vi "P-733 Control.vi"(0 "P-733 Notifier":refnum<notifier>, 5 "Stage Actions":T1={"Action"=enum."Get Position", "Axis"=[], "Setpoint"=[], "Velocity"=0.5, "Cmd Recvd?"=FALSE, "Position"=[], "Status"=enum."Error", "Misc"=variant} {"Velocity" min=0.0 max=1.0 step=0.01}, 11 "VISA In":refnum<visa-resource-name>, 13 "Axis Names":string[](array[string])) -> (4 "P-612 Notifier (Dup)":refnum<notifier>)   [LabVIEW 2016]
uses:
  Stages Controls/Stage Notifier Element.ctl
  Stages Controls/Stage Actions.ctl
  Stages Controls/Stage Status.ctl
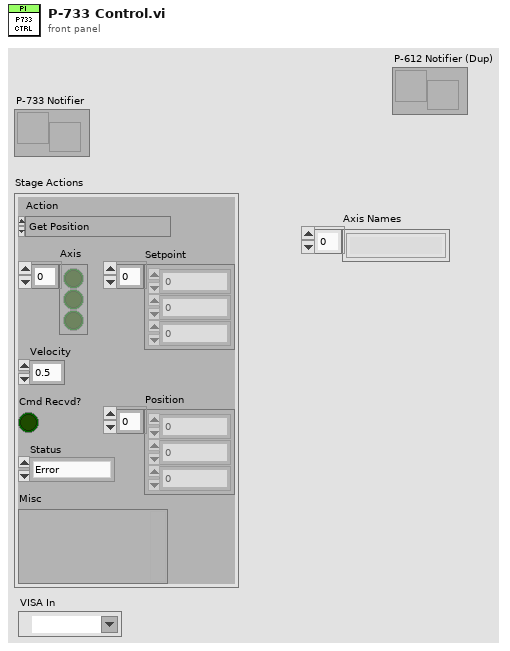
[diagram p1: front panel]
types:
  T1 = typedef "Stage Notifier Element.ctl" = cluster{"Action":T2, "Axis":bool[], "Setpoint":dbl[], "Velocity":dbl, "Cmd Recvd?":bool, "Position":dbl[], "Status":T3, "Misc":variant}
  T2 = typedef "Stage Actions.ctl" = enum16{"Get Position", "MVR", "MOVE", "HALT", "ONTARGET", "ERROR", "REFERENCE", "INIT", "VELOCITY", "STATUS", "EXIT", "HOME", "ZEROPOS", "NANOPOS", "ANALOG", "QUIT"}
  T3 = typedef "Stage Status.ctl" = enum16{"Error", "Abort", "Busy", "On Target"}
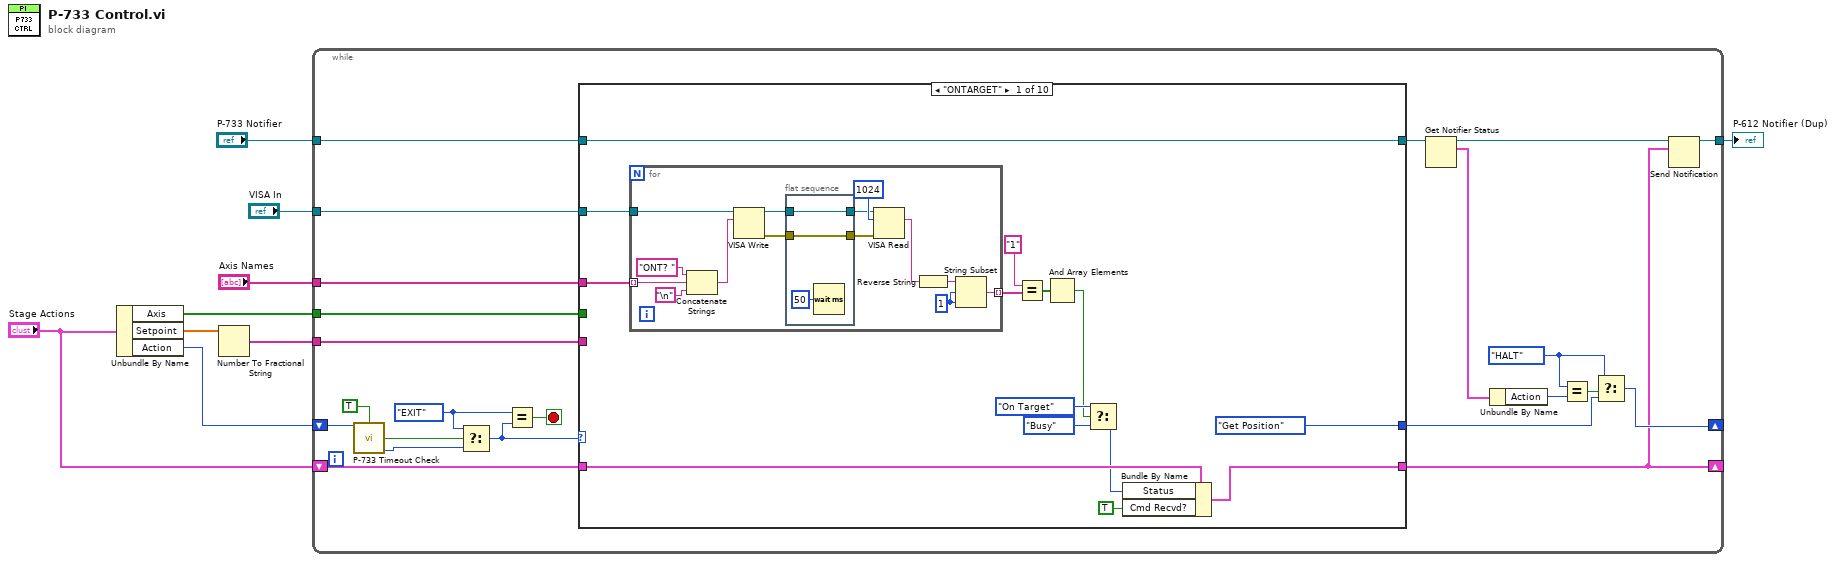
[diagram p0: block diagram]
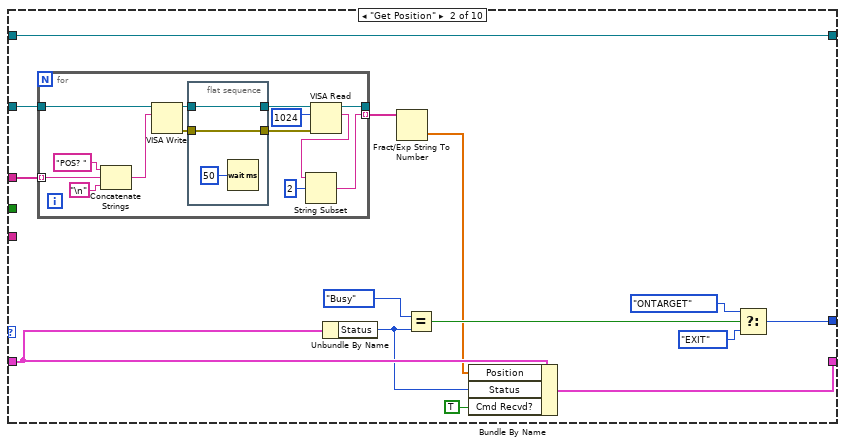
[diagram p2: hidden frame]
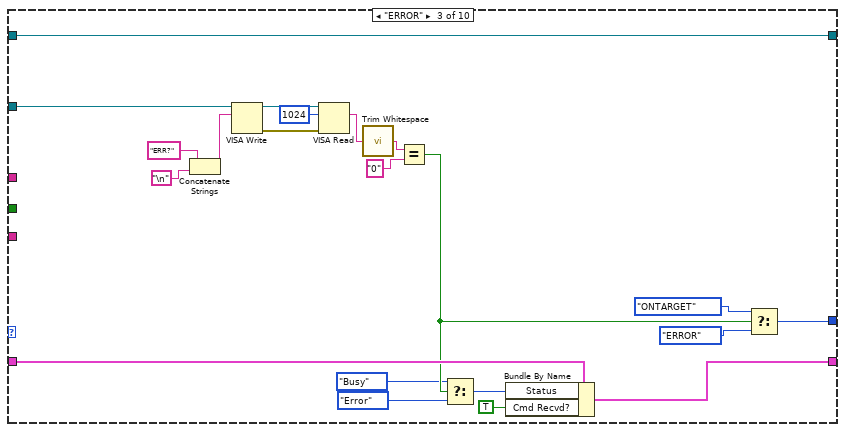
[diagram p3: hidden frame]
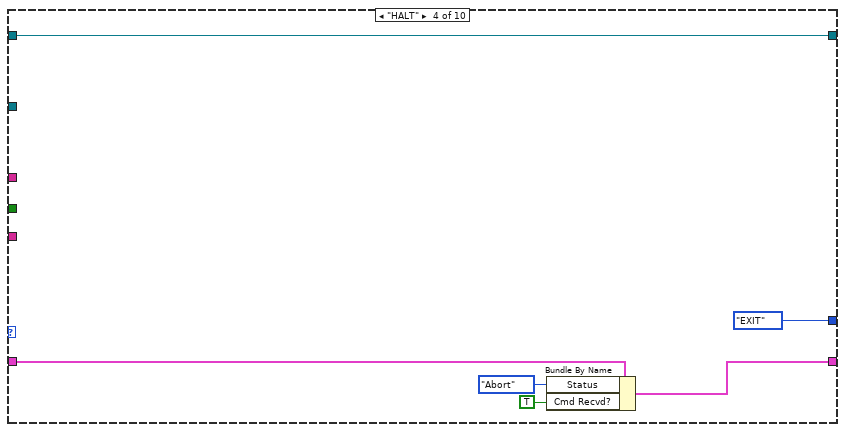
[diagram p4: hidden frame]
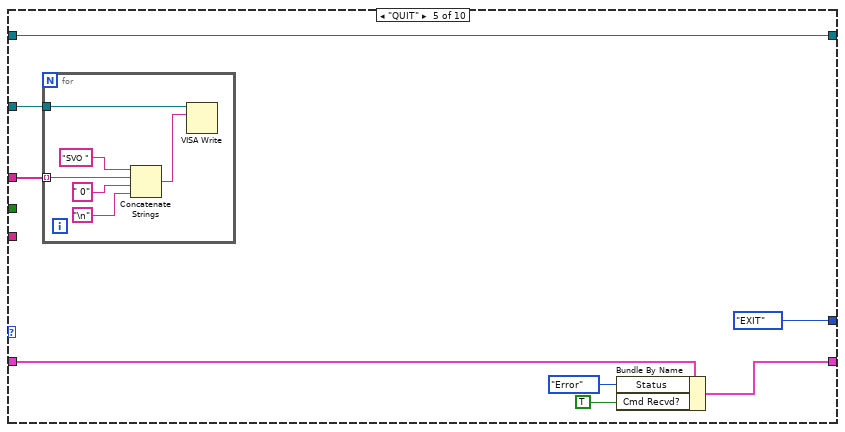
[diagram p5: hidden frame]
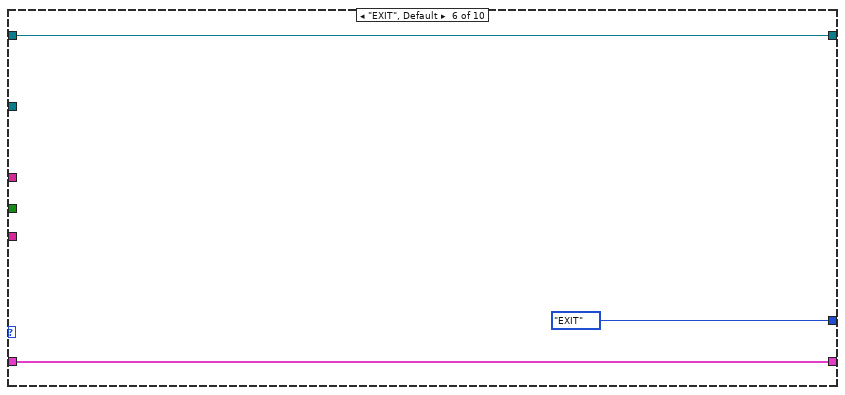
[diagram p6: hidden frame]
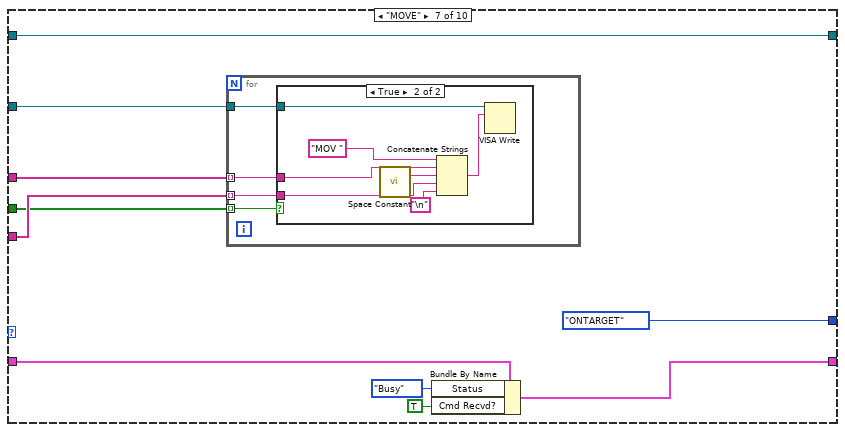
[diagram p7: hidden frame]
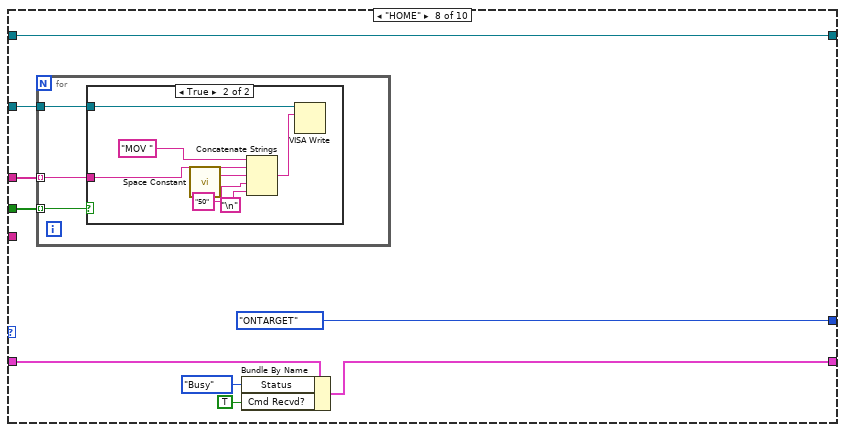
[diagram p9: hidden frame]
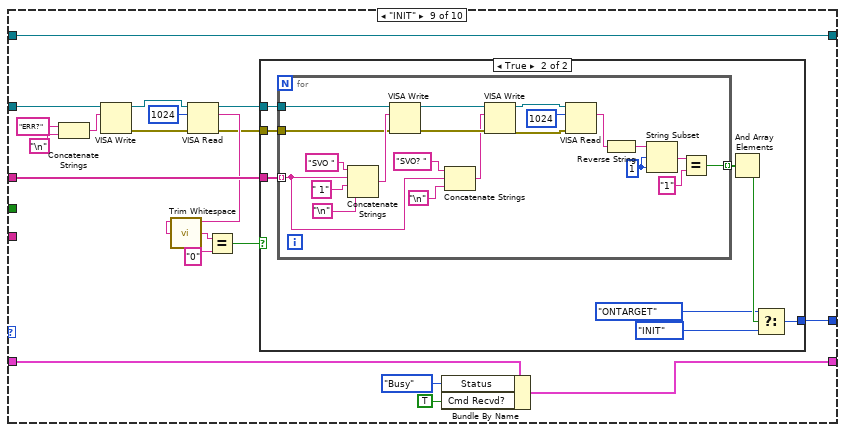
[diagram p11: hidden frame]
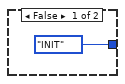
[diagram p12: hidden frame]
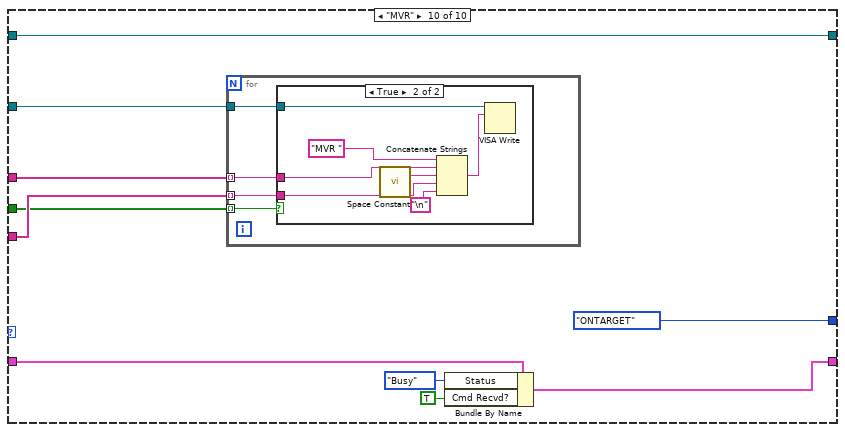
[diagram p13: hidden frame]
diagram:
  n1 = Unbundle By Name("Stage Actions") -> ("Axis"=w8:bool[], "Setpoint"=w7:dbl[], "Action"=w6:T2)
  n2 = Number To Fractional String(number=w7) -> (F-format string=w9:string[])  [unwired: 3 in]
  n3 = while {
    tunnel: "Axis Names" -> [w32]
    shift-right: [w27] -> _
    shift-left: w6 -> [w24]
    tunnel: w8 -> [w30]
    tunnel: w9 -> [w31]
    shift-right: [w26] -> _
    shift-left: "Stage Actions" -> [w29]
    tunnel: "P-733 Notifier" -> [w18]
    tunnel: "VISA In" -> [w17]
    tunnel: [w10] -> w2
    stop <- w19 stop-if-true
    w13 = Stage_Actions."HALT" ("Action")
    w23 = Stage_Actions."EXIT" ("t")
    n4 = call "P-733 Timeout Check.vi"("Action"=w24, "User Input?"=TRUE) -> ("Timeout?"=w22:bool, "Action (Dup)"=w21:T2)  [unwired: 12 in]
    n5 = Select(t=w23, s=w22, f=w21) -> (s? t:f=w20:T2)
    n6 = Equal?(x=w23, y=w20) -> (x = y?=w19:bool)
    n7 = case shown="\"ONTARGET\"" w20 {
      tunnel: w32 -> [w46 w77 _ _ w128 _ w148 w168 w198 w238]
      tunnel: w31 -> [_ _ _ _ _ _ w147 _ _ w237]
      tunnel: w30 -> [_ _ _ _ _ _ w146 w167 _ w236]
      tunnel: [Stage_Actions."Get Position" ("y") w75 w104 Stage_Actions."EXIT" ("y") Stage_Actions."EXIT" ("y") Stage_Actions."EXIT" ("y") Stage_Actions."ONTARGET" ("y") Stage_Actions."ONTARGET" ("y") w193 Stage_Actions."ONTARGET" ("y")] -> w28
      tunnel: w29 -> [w40 w73 w99 w117 w126 w138 w143 w164 w195 w233]
      tunnel: [w41 w70 w100 w118 w125 w138 w142 w163 w194 w232] -> w26
      tunnel: w18 -> [w34 w64 w95 w116 w122 w136 w139 w161 w179 w229]
      tunnel: [w34 w64 w95 w116 w122 w136 w139 w161 w179 w229] -> w11
      tunnel: w17 -> [w33 w65 w96 _ w123 _ w140 w160 w180 w230]
      frame "ONTARGET" {
        n8 = for {
          tunnel: w46 -> [w60] mode=indexing
          tunnel: [w59] -> w45 mode=indexing
          tunnel: w33 -> [w47]
          w54 = 1 ("length (rest)")
          n9 = Concatenate Strings("ONT? " ("string"), w60, "\n") -> (w53:string)
          n10 = VISA Write(VISA resource name=w47, write buffer=w53) -> (VISA resource name out=w50:refnum<visa-resource-name>, error out=w48:errorcluster)  [unwired: 1 in, 1 out]
          n11 = flat-sequence {
            tunnel: [w63] -> w51
            tunnel: w50 -> [w63]
            tunnel: [w62] -> w49
            tunnel: w48 -> [w62]
            frame #0 {
              n12 = Wait (ms)(milliseconds to wait=u32 50) -> ()  [unwired: 1 out]
            }
          }
          n13 = VISA Read(VISA resource name=w51, byte count=u32 1024, error in (no error)=w49) -> (read buffer=w52:string)  [unwired: 3 out]
          n14 = Reverse String(1:w52) -> (0:w55:string)
          n15 = String Subset(string=w55, offset (0)=w54, length (rest)=w54) -> (substring=w59:string)
        }
        n16 = Equal?(x="1", y=w45) -> (x = y?=w43:bool[])
        n17 = And Array Elements(Boolean array=w43) -> (logical AND=w37:bool)
        n18 = Select(t=Stage_Status."On Target" ("Status"), s=w37, f=Stage_Status."Busy" ("Status")) -> (s? t:f=w36:T3)
        n19 = Bundle By Name(cluster=w40, "Status"=w36, "Cmd Recvd?"=TRUE) -> (w41:T1)
      }
      frame "Get Position" {
        n20 = for {
          tunnel: w77 -> [w91] mode=indexing
          tunnel: [w80] -> w76 mode=indexing
          tunnel: [w82] -> _
          tunnel: w65 -> [w81]
          n21 = Concatenate Strings("POS? " ("string"), w91, "\n") -> (w87:string)
          n22 = VISA Write(VISA resource name=w81, write buffer=w87) -> (VISA resource name out=w85:refnum<visa-resource-name>, error out=w83:errorcluster)  [unwired: 1 in, 1 out]
          n23 = flat-sequence {
            tunnel: [w94] -> w86
            tunnel: w85 -> [w94]
            tunnel: [w93] -> w84
            tunnel: w83 -> [w93]
            frame #0 {
              n24 = Wait (ms)(milliseconds to wait=u32 50) -> ()  [unwired: 1 out]
            }
          }
          n25 = VISA Read(VISA resource name=w86, byte count=u32 1024, error in (no error)=w84) -> (VISA resource name out=w82:refnum<visa-resource-name>, read buffer=w79:string)  [unwired: 2 out]
          n26 = String Subset(string=w79, offset (0)=2) -> (substring=w80:string)  [unwired: 1 in]
        }
        n27 = Unbundle By Name(w73) -> ("Status"=w68:T3)
        n28 = Fract/Exp String To Number(string=w76) -> (number=w69:dbl[])  [unwired: 3 in, 1 out]
        n29 = Equal?(x=Stage_Status."Busy", y=w68) -> (x = y?=w71:bool)
        n30 = Bundle By Name(cluster=w73, "Position"=w69, "Status"=w68, "Cmd Recvd?"=TRUE) -> (w70:T1)
        n31 = Select(t=Stage_Actions."ONTARGET" ("y"), s=w71, f=Stage_Actions."EXIT" ("y")) -> (s? t:f=w75:T2)
      }
      frame "ERROR" {
        n32 = Concatenate Strings("ERR?" ("string"), "\n") -> (w108:string)
        n33 = VISA Write(VISA resource name=w96, write buffer=w108) -> (VISA resource name out=w107:refnum<visa-resource-name>, error out=w112:errorcluster)  [unwired: 1 in, 1 out]
        n34 = VISA Read(VISA resource name=w107, byte count=u32 1024, error in (no error)=w112) -> (read buffer=w113:string)  [unwired: 3 out]
        n35 = call <vilib>:"Trim Whitespace.vi"("string"=w113) -> ("trimmed string"=w115:string)  [unwired: 1 in]
        n36 = Equal?(x=w115, y="0") -> (x = y?=w98:bool)
        n37 = Select(t=Stage_Status."Busy" ("Status"), s=w98, f=Stage_Status."Error" ("Status")) -> (s? t:f=w102:T3)
        n38 = Bundle By Name(cluster=w99, "Status"=w102, "Cmd Recvd?"=TRUE) -> (w100:T1)
        n39 = Select(t=Stage_Actions."ONTARGET" ("Action"), s=w98, f=Stage_Actions."ERROR") -> (s? t:f=w104:T2)
      }
      frame "HALT" {
        n40 = Bundle By Name(cluster=w117, "Status"=Stage_Status."Abort", "Cmd Recvd?"=TRUE) -> (w118:T1)
      }
      frame "QUIT" {
        n41 = for {
          tunnel: w128 -> [w132] mode=indexing
          tunnel: w123 -> [w130]
          n42 = Concatenate Strings("SVO " ("write buffer"), w132, " 0" ("string"), "\n") -> (w131:string)
          n43 = VISA Write(VISA resource name=w130, write buffer=w131) -> ()  [unwired: 1 in, 3 out]
        }
        n44 = Bundle By Name(cluster=w126, "Status"=Stage_Status."Error", "Cmd Recvd?"=TRUE) -> (w125:T1)
      }
      frame "EXIT", Default {
      }
      frame "MOVE" {
        n45 = for {
          tunnel: w148 -> [w152] mode=indexing
          tunnel: w147 -> [w151] mode=indexing
          tunnel: w146 -> [w150] mode=indexing
          tunnel: w140 -> [w149]
          n46 = case shown="True" w150 {
            tunnel: w152 -> [_ w157]
            tunnel: w151 -> [_ w154]
            tunnel: w149 -> [_ w153]
            frame False {
            }
            frame True {
              n47 = call <vilib>:"Space Constant.vi"() -> ("String"=w155:string)
              n48 = Concatenate Strings("MOV ", w157, w155, w154, "\n") -> (w159:string)
              n49 = VISA Write(VISA resource name=w153, write buffer=w159) -> ()  [unwired: 1 in, 3 out]
            }
          }
        }
        n50 = Bundle By Name(cluster=w143, "Status"=Stage_Status."Busy", "Cmd Recvd?"=TRUE) -> (w142:T1)
      }
      frame "HOME" {
        n51 = for {
          tunnel: w168 -> [w171] mode=indexing
          tunnel: w167 -> [w170] mode=indexing
          tunnel: w160 -> [w169]
          n52 = case shown="True" w170 {
            tunnel: w171 -> [_ w176]
            tunnel: w169 -> [_ w172]
            frame False {
            }
            frame True {
              n53 = call <vilib>:"Space Constant.vi"() -> ("String"=w174:string)
              n54 = Concatenate Strings("MOV ", w176, w174, "50" ("string"), "\n") -> (w178:string)
              n55 = VISA Write(VISA resource name=w172, write buffer=w178) -> ()  [unwired: 1 in, 3 out]
            }
          }
        }
        n56 = Bundle By Name(cluster=w164, "Status"=Stage_Status."Busy", "Cmd Recvd?"=TRUE) -> (w163:T1)
      }
      frame "INIT" {
        n57 = Concatenate Strings("ERR?" ("string"), "\n") -> (w190:string)
        n58 = VISA Write(VISA resource name=w180, write buffer=w190) -> (VISA resource name out=w185:refnum<visa-resource-name>, error out=w183:errorcluster)  [unwired: 1 in, 1 out]
        n59 = VISA Read(VISA resource name=w185, byte count=u32 1024, error in (no error)=w183) -> (VISA resource name out=w184:refnum<visa-resource-name>, read buffer=w187:string, error out=w182:errorcluster)  [unwired: 1 out]
        n60 = call <vilib>:"Trim Whitespace.vi"("string"=w187) -> ("trimmed string"=w189:string)  [unwired: 1 in]
        n61 = Equal?(x=w189, y="0") -> (x = y?=w181:bool)
        n62 = case shown="True" w181 {
          tunnel: w198 -> [_ w207]
          tunnel: [Stage_Actions."INIT" ("y") w203] -> w193
          tunnel: w184 -> [_ w200]
          tunnel: w182 -> [_ w201]
          frame False {
          }
          frame True {
            n63 = for {
              tunnel: w207 -> [w215] mode=indexing
              tunnel: [w212] -> w206 mode=indexing
              tunnel: w201 -> [w211]
              tunnel: w200 -> [w208]
              w224 = 1 ("length (rest)")
              n64 = Concatenate Strings("SVO " ("string"), w215, " 1" ("string"), "\n") -> (w216:string)
              n65 = VISA Write(VISA resource name=w208, write buffer=w216, error in (no error)=w211) -> (VISA resource name out=w210:refnum<visa-resource-name>, error out=w228:errorcluster)  [unwired: 1 out]
              n66 = Concatenate Strings("SVO? " ("string"), w215, "\n") -> (w214:string)
              n67 = VISA Write(VISA resource name=w210, write buffer=w214, error in (no error)=w228) -> (VISA resource name out=w209:refnum<visa-resource-name>, error out=w227:errorcluster)  [unwired: 1 out]
              n68 = VISA Read(VISA resource name=w209, byte count=u32 1024, error in (no error)=w227) -> (read buffer=w225:string)  [unwired: 3 out]
              n69 = Reverse String(1:w225) -> (0:w223:string)
              n70 = String Subset(string=w223, offset (0)=w224, length (rest)=w224) -> (substring=w226:string)
              n71 = Equal?(x=w226, y="1") -> (x = y?=w212:bool)
            }
            n72 = And Array Elements(Boolean array=w206) -> (logical AND=w205:bool)
            n73 = Select(t=Stage_Actions."ONTARGET" ("y"), s=w205, f=Stage_Actions."INIT" ("y")) -> (s? t:f=w203:T2)
          }
        }
        n74 = Bundle By Name(cluster=w195, "Status"=Stage_Status."Busy", "Cmd Recvd?"=TRUE) -> (w194:T1)
      }
      frame "MVR" {
        n75 = for {
          tunnel: w238 -> [w242] mode=indexing
          tunnel: w237 -> [w241] mode=indexing
          tunnel: w236 -> [w240] mode=indexing
          tunnel: w230 -> [w239]
          n76 = case shown="True" w240 {
            tunnel: w242 -> [_ w247]
            tunnel: w241 -> [_ w244]
            tunnel: w239 -> [_ w243]
            frame False {
            }
            frame True {
              n77 = call <vilib>:"Space Constant.vi"() -> ("String"=w245:string)
              n78 = Concatenate Strings("MVR ", w247, w245, w244, "\n") -> (w249:string)
              n79 = VISA Write(VISA resource name=w243, write buffer=w249) -> ()  [unwired: 1 in, 3 out]
            }
          }
        }
        n80 = Bundle By Name(cluster=w233, "Status"=Stage_Status."Busy", "Cmd Recvd?"=TRUE) -> (w232:T1)
      }
    }
    n81 = Get Notifier Status(notifier=w11) -> (notifier out=w16:refnum<notifier>, current notification=w12:T1)  [unwired: 1 in, 3 out]
    n82 = Unbundle By Name(w12) -> ("Action"=w14:T2)
    n83 = Equal?(x=w13, y=w14) -> (x = y?=w15:bool)
    n84 = Select(t=w13, s=w15, f=w28) -> (s? t:f=w27:T2)
    n85 = Send Notification(notification=w26, notifier=w16) -> (notifier out=w10:refnum<notifier>)  [unwired: 1 in, 1 out]
  }
  "P-612 Notifier (Dup)" <- w2
